vi "PRN Generation_Station_2.vi"(8 "error in (no error)":errorcluster, 10 "PRN path":path, 11 "Cluster":T2) -> (0 "error out":errorcluster, 1 "Barcode Station 2 Up":string, 2 "Barcode station 2 Dn":string, 3 "PRN to Print":string)   [LabVIEW 2017]
uses:
  <vilib>/addons/database/Connection.llb/Conn ObjectReference.ctl
  <vilib>/addons/database/NI_Database_API.lvlib
panel:
  out "appended array":string[](array[string])
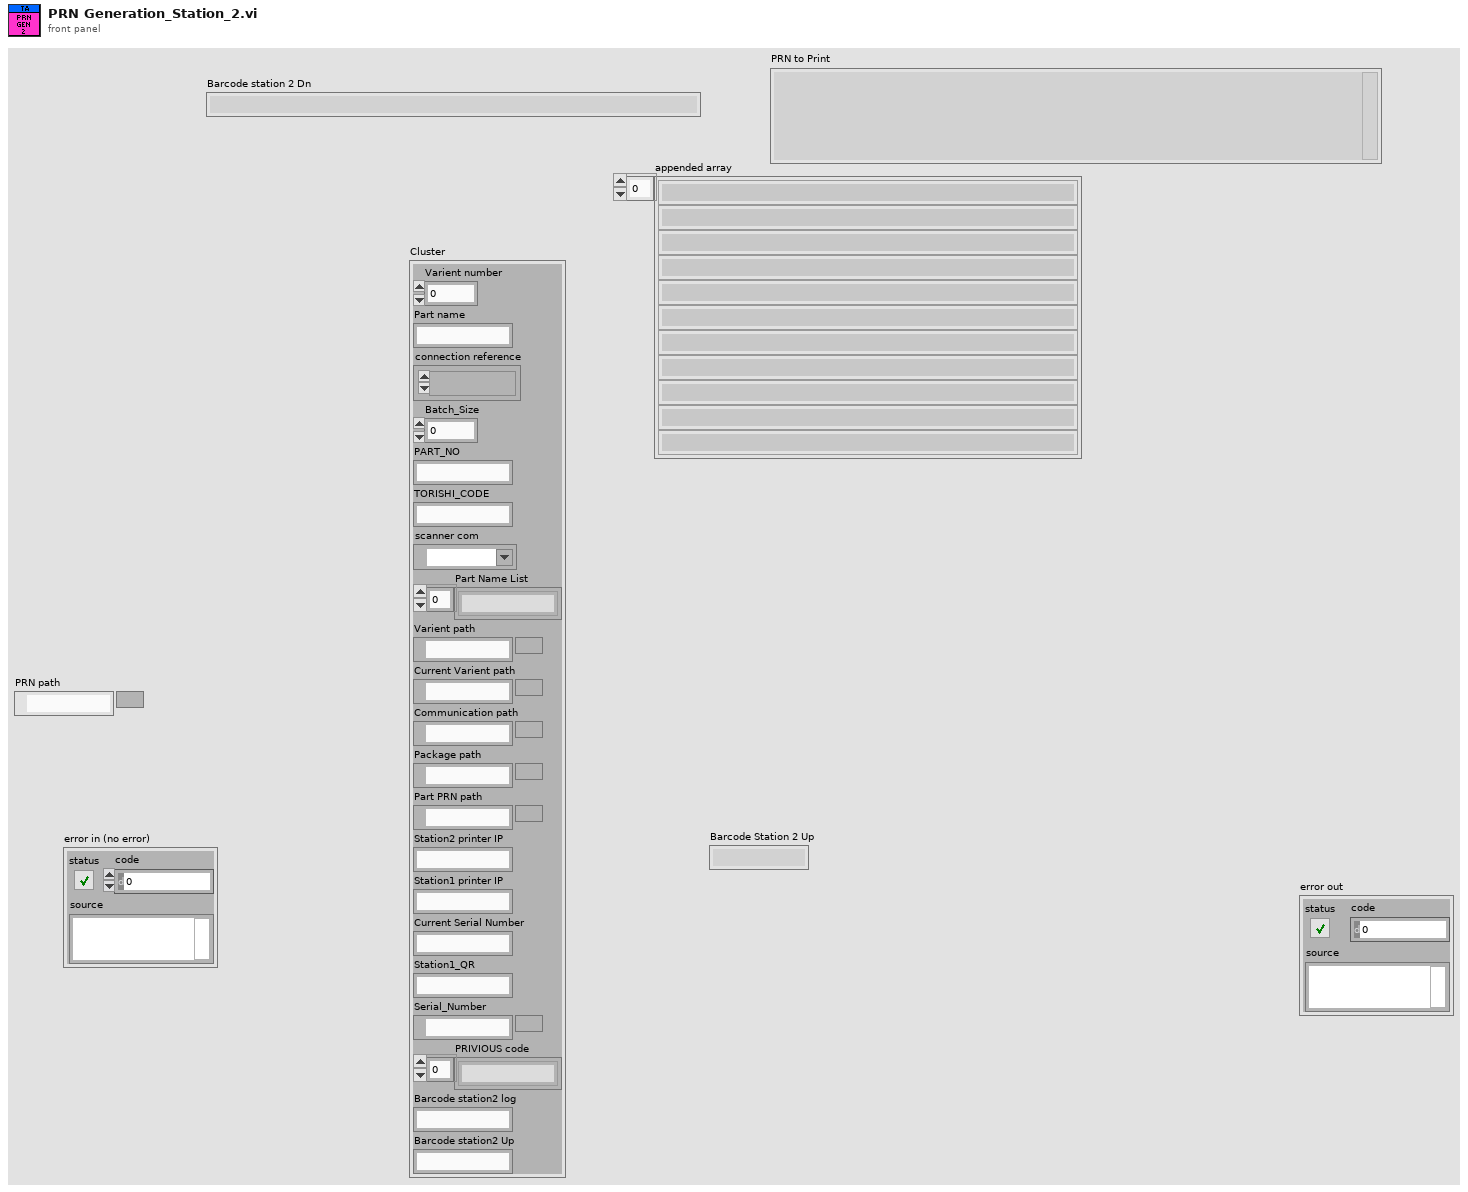
[diagram p1: front panel]
types:
  T1 = typedef "NI_Database_API.lvlib/Conn ObjectReference.ctl" = refnum<k1>
  T2 = cluster{"Varient number":u16, "Part name":string, "connection reference":T1, "Batch_Size":u16, "PART_NO":string, "TORISHI_CODE":string, "scanner com":refnum<visa-resource-name>, "Part Name List":string[], "Varient path":path, "Current Varient path":path, "Communication path":path, "Package path":path, "Part PRN path":path, "Station2 printer IP":string, "Station1 printer IP":string, "Current Serial Number":string, "Station1_QR":string, "Serial_Number":path, "PRIVIOUS code":string[], "Barcode station2 log":string, "Barcode station2 Up":string}
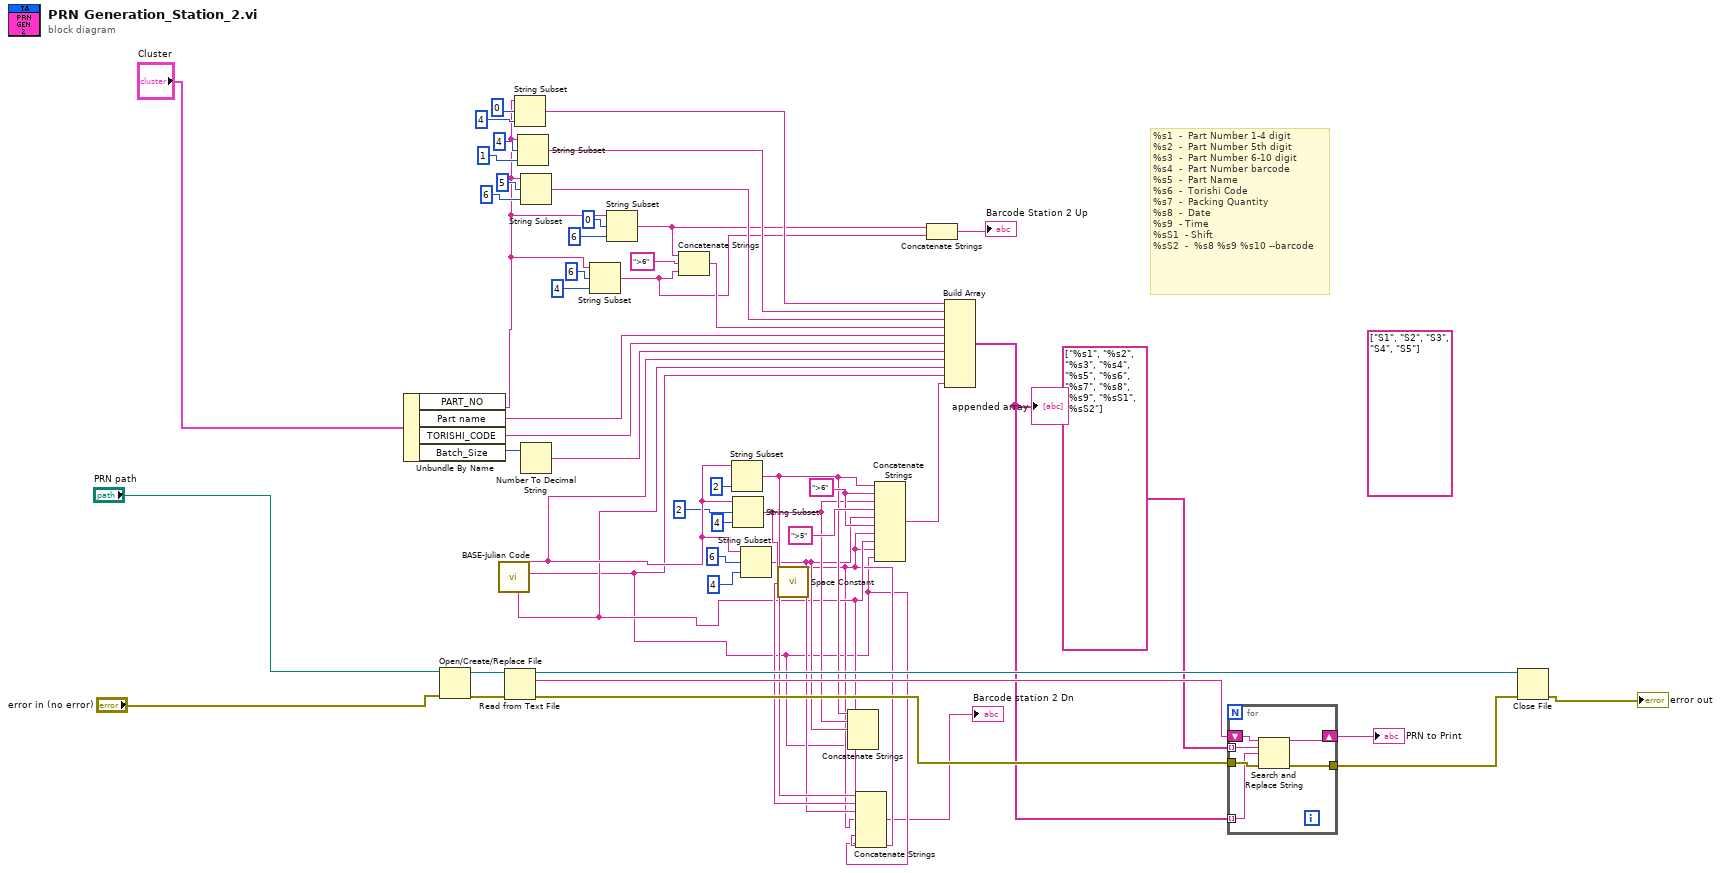
[diagram p0: block diagram]
diagram:
  w21 = ">6" ("string")
  (unwired) string[] ["S1", "S2", "S3", "S4", "S5"]
  # "%s1  -  Part Number 1-4 digit\n%s2  -  Part Number 5th digit\n%s3  -  Part Number 6-10 digit\n%s4  -  Part Number barcode\n%s5  -  Part Name\n%s6  -  Torishi Code\n%s7  -  Packing Quantity\n%s8  -  Date\n%s9  - Time\n%sS1  - Shift\n%sS2  -  %s8 %s9 %s10 --barcode"
  n1 = Unbundle By Name("Cluster") -> ("PART_NO"=w13:string, "Part name"=w31:string, "TORISHI_CODE"=w30:string, "Batch_Size"=w42:u16)
  n2 = Open/Create/Replace File(file path (use dialog)="PRN path", error in="error in (no error)") -> (refnum out=w49:refnum<file>, error out=w50:errorcluster)  [unwired: 4 in, 1 out]
  n3 = call "BASE-Julian Code.vi"() -> ("Shift"=w2:string, "Long time with :"=w4:string, "Long date with /"=w23:string)  [unwired: 6 in, 3 out]
  n4 = Read from Text File(file (use dialog)=w49, error in=w50) -> (refnum out=w51:refnum<file>, text=w47:string, error out=w45:errorcluster)  [unwired: 2 in, 1 out]
  n5 = String Subset(string=w13, offset (0)=0, length (rest)=4 ("length (rest)")) -> (substring=w34:string)
  n6 = String Subset(string=w13, offset (0)=4, length (rest)=1 ("length (rest)")) -> (substring=w33:string)
  n7 = String Subset(string=w13, offset (0)=5, length (rest)=6 ("length (rest)")) -> (substring=w32:string)
  n8 = Number To Decimal String(number=w42) -> (decimal integer string=w29:string)  [unwired: 1 in]
  n9 = String Subset(string=w13, offset (0)=6, length (rest)=4 ("length (rest)")) -> (substring=w9:string)
  n10 = String Subset(string=w13, offset (0)=0, length (rest)=6 ("length (rest)")) -> (substring=w10:string)
  n11 = Concatenate Strings(w10, ">6" ("string"), w9) -> (w12:string)
  n12 = String Subset(string=w23, length (rest)=2 ("length (rest)")) -> (substring=w7:string)  [unwired: 1 in]
  n13 = String Subset(string=w23, offset (0)=2, length (rest)=4 ("length (rest)")) -> (substring=w6:string)
  n14 = String Subset(string=w23, offset (0)=6, length (rest)=4 ("length (rest)")) -> (substring=w5:string)
  n15 = call <vilib>:"Space Constant.vi"() -> ("String"=w3:string)
  n16 = Concatenate Strings(w7, w6, w5, w4, w2) -> ()  [unwired: 1 out]
  n17 = Concatenate Strings(w7, w6, w5, w3, w4, w3, w2) -> (→"Barcode station 2 Dn":string)
  n18 = Concatenate Strings(w7, w21, w6, ">5" ("string"), w5, w21, w3, w4, w3, w2) -> (w20:string)
  n19 = Concatenate Strings(w10, w9) -> (→"Barcode Station 2 Up":string)
  n20 = Build Array(w34, w33, w32, w12, w31, w30, w29, w23, w4, w2, w20) -> (w28:string[])
  "appended array" <- w28
  n21 = for {
    shift-right: [w57] -> w46
    shift-left: w47 -> [w58]
    tunnel: w45 -> [w56]
    tunnel: [w55] -> w44
    tunnel: string[] ["%s1", "%s2", "%s3", "%s4", "%s5", "%s6", "%s7", "%s8", "%s9", "%sS1", "%sS2"] -> [w54] mode=indexing
    tunnel: w28 -> [w53] mode=indexing
    n22 = Search and Replace String(input string=w58, search string=w54, replace string=w53, error in=w56) -> (result string=w57:string, error out=w55:errorcluster)  [unwired: 4 in, 2 out]
  }
  "PRN to Print" <- w46
  n23 = Close File(refnum=w51, error in=w44) -> (error out=→"error out":errorcluster)  [unwired: 1 out]
